vi "SET_AP_CH&DC_OFF.vi"(0 "Frequency (Hz)":dbl=100000.0 format="%#_6f", 1 "VISA_SGEN":refnum<visa-resource-name>="GPIB0::30::INSTR", 2 "Enable Output (T: Enable)":bool, 5 "CHA Amp (V)":dbl=3.491 format="%_4g", 9 "DC Offset (0 V)":dbl=1.795, 11 "error in (no error)":errorcluster) -> (15 "error out":errorcluster)   [LabVIEW 2019]
uses:
  <userlib>/_TI-LA/Instr Drivers/Audio Analyzer/AP27xx/Modules/Common/AP27xx Application Settings.ctl
  <userlib>/_TI-LA/Instr Drivers/Audio Analyzer/AP27xx/Driver/EasyIO/Analog Generator/Typedefs/AP27xx_Analog Generator Waveform Type.ctl
  <userlib>/_TI-LA/Instr Drivers/Audio Analyzer/AP27xx/Driver/EasyIO/Analog Generator/Typedefs/AP27xx_Analog Generator Waveform Setting.ctl
  <userlib>/_TI-LA/Instr Drivers/Audio Analyzer/AP27xx/Driver/EasyIO/Common/Typedefs/AP27xx_Frequency Units.ctl
  <userlib>/_TI-LA/Instr Drivers/Audio Analyzer/AP27xx/Driver/EasyIO/Analog Generator/Typedefs/AP27xx_Analog Generator Amplitude Units.ctl
  <userlib>/_TI-LA/Instr Drivers/Audio Analyzer/AP27xx/Driver/EasyIO/Analog Generator/Typedefs/AP27xx_Analog Generator Freq Accuracy.ctl
  <userlib>/_TI-LA/Instr Drivers/Audio Analyzer/AP27xx/Driver/EasyIO/Analog Generator/Typedefs/AP27xx_Analog Generator Waveform Configuration.ctl
  <userlib>/_TI-LA/Instr Drivers/Audio Analyzer/AP27xx/Driver/EasyIO/Analog Generator/Typedefs/AP27xx_Analog Generator Waveform Impedance.ctl
  <userlib>/_TI-LA/Instr Drivers/Audio Analyzer/AP27xx/Driver/EasyIO/Analog Generator/Typedefs/AP27xx_Analog Generator Waveform Impedance (unbal).ctl
  <userlib>/_TI-LA/Instr Drivers/Audio Analyzer/AP27xx/Driver/EasyIO/Analog Generator/Typedefs/AP27xx_Analog Generator Waveform DAC Bandwidth.ctl
  <userlib>/_TI-LA/Instr Drivers/Audio Analyzer/AP27xx/Driver/EasyIO/Analog Generator/Typedefs/AP27xx_Analog Generator Output Setting.ctl
  <userlib>/_TI-LA/Instr Drivers/Audio Analyzer/AP27xx/Driver/EasyIO/Analog Generator/Typedefs/AP27xx_Analog Generator Reference Setting.ctl
  <userlib>/_TI-LA/Instr Drivers/Power Supply/E3631/Driver/EasyIO/Typedefs/E3631 Outputs Settings.ctl
  <userlib>/_TI-LA/Instr Drivers/Power Supply/E3631/Driver/EasyIO/Typedefs/E3631 Output Configuration.ctl
  <userlib>/_TI-LA/Instr Drivers/Power Supply/E3631/Driver/EasyIO/Typedefs/E3631 Action.ctl
  <userlib>/_TI-LA/Instr Drivers/Power Supply/E3631/Driver/EasyIO/Typedefs/E3631 OP State.ctl
  <userlib>/_TI-LA/Instr Drivers/Audio Analyzer/AP27xx/Modules/AP27xx Modules.lvlib
  <userlib>/_TI-LA/Instr Drivers/Audio Analyzer/AP27xx/Driver/EasyIO/Analog Generator/AP27xx Analog Generator.lvlib
  <userlib>/_TI-LA/Instr Drivers/Audio Analyzer/AP27xx/Driver/EasyIO/Common/AP27xx Common.lvlib
  <userlib>/_TI-LA/Instr Drivers/Power Supply/E3631/Driver/E3631.lvlib
panel:
  in  "f_In":dbl format="%#_13g"
  # "3.491"
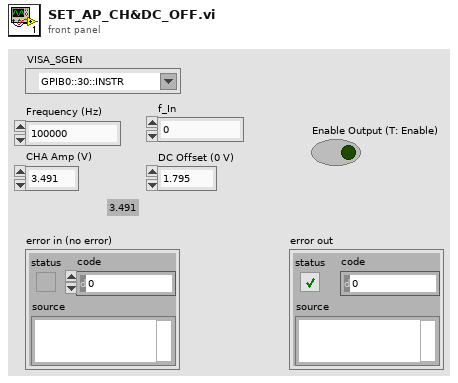
[diagram p1: front panel]
types:
  T1 = typedef "E3631.lvlib/E3631 Outputs Settings.ctl" = cluster{"Channel 1 (+6V)":T2, "Channel 2 (+25V)":T2, "Channel 3 (-25V)":T2}
  T2 = typedef "E3631.lvlib/E3631 Output Configuration.ctl" = cluster{"action":T3, "voltage (V)":dbl, "current limit (A)":dbl, "Enable?":bool}
  T3 = typedef "E3631.lvlib/E3631 Action.ctl" = enum16{"Configure channel", "Keep current settings"}
  T4 = typedef "AP27xx Analog Generator.lvlib/AP27xx_Analog Generator Reference Setting.ctl" = cluster{"dBm (Ohm)":dbl, "Freq (Hz)":dbl, "dBr (Vrms)":dbl, "Watts (Ohm)":dbl}
  T5 = typedef "AP27xx Analog Generator.lvlib/AP27xx_Analog Generator Output Setting.ctl" = cluster{"Outputs":bool, "Auto ON":bool, "CHA invert":bool, "CHA output":bool, "CHB invert":bool, "CHB output":bool, "Track A":bool}
  T6 = typedef "AP27xx Analog Generator.lvlib/AP27xx_Analog Generator Waveform Setting.ctl" = cluster{"Frequency Unit":T7, "Frequency (Hz)":dbl, "CHA Amp Unit":T8, "CHA Amp (V)":dbl, "Freq accuracy":T9, "CHB Amp (V)":dbl, "Configuration":T10, "Impedance (bal & CMTST)":T11, "Impedance (unbal)":T12, "DAC Bandwidth":T13, "CHB Amp Unit":T8}
  T7 = typedef "AP27xx Common.lvlib/AP27xx_Frequency Units.ctl" = enum16{"Hz", "F/R", "dHz", "%Hz", "cent", "octs", "decs", " d%", "dPPM"}
  T8 = typedef "AP27xx Analog Generator.lvlib/AP27xx_Analog Generator Amplitude Units.ctl" = enum16{"Vrms", "Vp", "Vpp", "dBu", "dBV", "dBr", "dBm", "W", "dBrInv"}
  T9 = typedef "AP27xx Analog Generator.lvlib/AP27xx_Analog Generator Freq Accuracy.ctl" = enum16{"Fast", "High accuracy"}
  T10 = typedef "AP27xx Analog Generator.lvlib/AP27xx_Analog Generator Waveform Configuration.ctl" = enum16{"Bal-Float", "Bal-Gnd", "Unbal-Float", "Unbal-Gnd", "CMTST"}
  T11 = typedef "AP27xx Analog Generator.lvlib/AP27xx_Analog Generator Waveform Impedance.ctl" = enum16{"40", "150", "600"}
  T12 = typedef "AP27xx Analog Generator.lvlib/AP27xx_Analog Generator Waveform Impedance (unbal).ctl" = enum16{"20", "600"}
  T13 = typedef "AP27xx Analog Generator.lvlib/AP27xx_Analog Generator Waveform DAC Bandwidth.ctl" = enum16{"30kHz (fs=65536)", "60kHz (fs=131072)"}
  T14 = typedef "AP27xx Analog Generator.lvlib/AP27xx_Analog Generator Waveform Type.ctl" = enum16{"Sine", "Sine (D/A)", "IMD", "IMD (D/A)", "Square", "Noise", "Arb Wfm (D/A)", "MLS (D/A)", "Special (D/A)", "Square (D/A)", "Noise (D/A)"}
  T15 = typedef "AP27xx Modules.lvlib/AP27xx Application Settings.ctl" = cluster{"Application Visible?":bool, "Quit APWin?":bool}
  T16 = typedef "E3631.lvlib/E3631 OP State.ctl" = enum16{"OFF", "ON"}
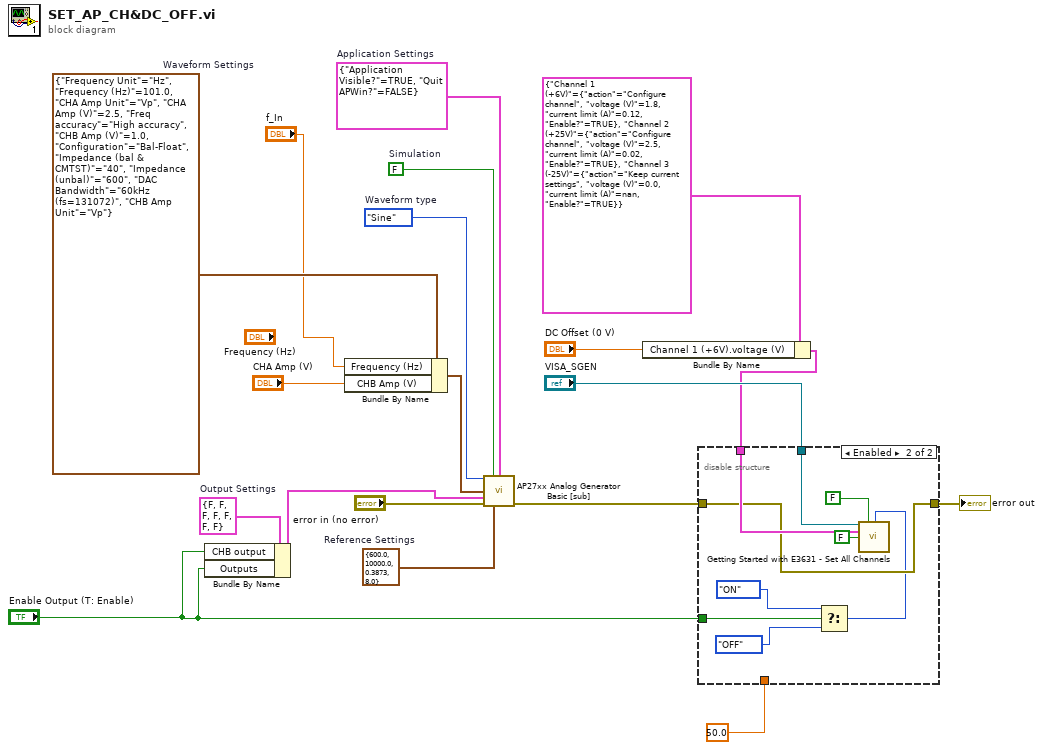
[diagram p0: block diagram]
diagram:
  w19 = T4 {"dBm (Ohm)"=600.0, "Freq (Hz)"=10000.0, "dBr (Vrms)"=0.3873, "Watts (Ohm)"=8.0}  # Reference Settings
  w8 = T5 {"Outputs"=FALSE, "Auto ON"=FALSE, "CHA invert"=FALSE, "CHA output"=FALSE, "CHB invert"=FALSE, "CHB output"=FALSE, "Track A"=FALSE}  # Output Settings
  w15 = T6 {"Frequency Unit"=enum."Hz", "Frequency (Hz)"=101.0, "CHA Amp Unit"=enum."Vp", "CHA Amp (V)"=2.5, "Freq accuracy"=enum."High accuracy", "CHB Amp (V)"=1.0, "Configuration"=enum."Bal-Float", "Impedance (bal & CMTST)"=enum."40", "Impedance (unbal)"=enum."600", "DAC Bandwidth"=enum."60kHz (fs=131072)", "CHB Amp Unit"=enum."Vp"}  # Waveform Settings
  w17 = AP27xx_Analog_Generator_Waveform_Type."Sine"  # Waveform type
  w16 = FALSE  # Simulation
  w18 = T15 {"Application Visible?"=TRUE, "Quit APWin?"=FALSE}  # Application Settings
  n1 = Bundle By Name(cluster=w8, "CHB output"="Enable Output (T: Enable)", "Outputs"="Enable Output (T: Enable)") -> (w7:T5)
  n2 = Bundle By Name(cluster=w15, "Frequency (Hz)"="f_In", "CHB Amp (V)"="CHA Amp (V)") -> (w14:T6)
  n3 = call <userlib>:"AP27xx Analog Generator Basic [sub].vi"("Waveform type"=w17, "Simulation"=w16, "Application Settings"=w18, "Waveform Settings"=w14, "Output Settings"=w7, "error in"="error in (no error)", "Reference Settings"=w19) -> ("error out"=w10:errorcluster)  [unwired: 8 in]
  n4 = Bundle By Name(cluster=T1 {"Channel 1 (+6V)"={"action"=enum."Configure channel", "voltage (V)"=1.8, "current limit (A)"=0.12, "Enable?"=TRUE}, "Channel 2 (+25V)"={"action"=enum."Configure channel", "voltage (V)"=2.5, "current limit (A)"=0.02, "Enable?"=TRUE}, "Channel 3 (-25V)"={"action"=enum."Keep current settings", "voltage (V)"=0.0, "current limit (A)"=nan, "Enable?"=TRUE}} ("E363x outputs settings"), "Channel 1 (+6V).voltage (V)"="DC Offset (0 V)") -> (w3:T1)
  n5 = disable-structure shown="Enabled" {
    disable-tunnel: "VISA_SGEN" -> [_ w29]
    disable-tunnel: w10 -> [w20 w27]
    disable-tunnel: [w20 w27] -> w9
    disable-tunnel: "Enable Output (T: Enable)" -> [_ w22]
    disable-tunnel: 50.0 ("Output Impedance (50 Ohm)") -> [_ _]
    disable-tunnel: w3 -> [_ w28]
    frame Disabled {
    }
    frame Enabled {
      n6 = Select(t=E3631_OP_State."ON" ("output state"), s=w22, f=E3631_OP_State."OFF" ("output state")) -> (s? t:f=w25:T16)
      n7 = call <userlib>:"Getting Started with E3631 - Set All Channels.vi"("Instrument handle In"=w29, "Reset"=FALSE, "output state"=w25, "E363x outputs settings"=w28, "Read Output?"=FALSE) -> ()  [unwired: 10 in, 1 out]
    }
  }
  "error out" <- w9
